vi "Create.vi"(8 "error in (no error)":errorcluster, 10 "UDP_Config":refnum<class "UDP_Config.lvclass">, 11 "UDP_Comm_Factory in":refnum<class "UDP_Comm_Factory.lvclass">) -> (0 "error out":errorcluster, 3 "UDP_Comm_Factory out":refnum<class "UDP_Comm_Factory.lvclass">)   [LabVIEW 2021, in "UDP_Comm_Factory.lvclass"]
uses:
  UDP_Comm_Factory.lvclass
  UDP_Config/UDP_Config.lvclass
  UDP_Sender/UDP_Sender.lvclass
  UDP_Receiver/UDP_Receiver.lvclass
  <vilib>/Utility/tcp.llb/UDP Multicast Write-Only Open.vi
  D:/Repository/UDP_Multicast/UDP_Comm/UDP_Comm.lvclass
  D:/Repository/UDP_Multicast/UDP_Sender/UDP_Sender.lvclass
  D:/Repository/UDP_Multicast/UDP_Receiver/UDP_Receiver.lvclass
  UDP_Comm/UDP_Comm.lvclass
panel:
  out "UDP_Comm":refnum<class "UDP_Comm.lvclass">
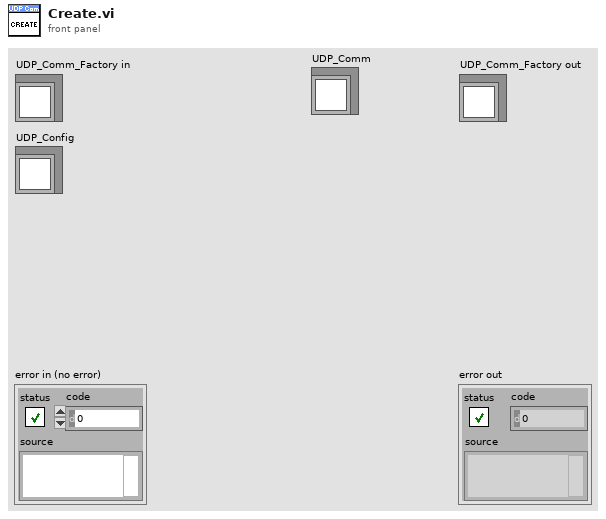
[diagram p1: front panel]
types:
  T1 = typedef "Role.ctl" = enum16{"Undefined", "Sender", "Receiver"}
  T2 = typedef "Network.ctl" = cluster{"MulticastGroup":string, "Port":u16, "LocalInterface":string, "TTL":u8}
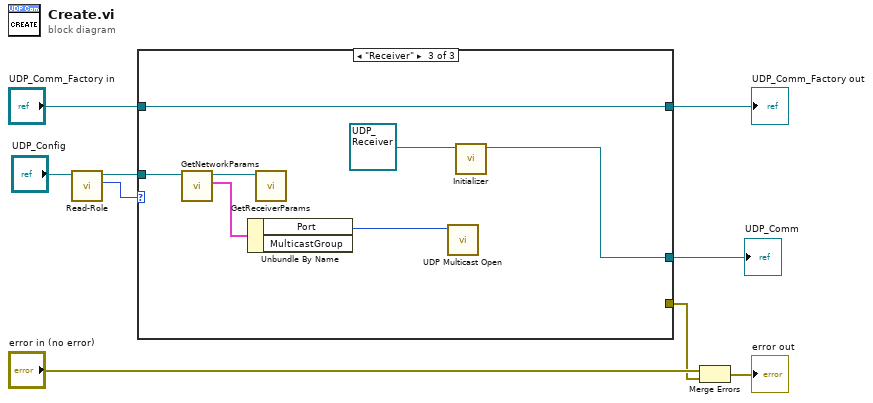
[diagram p0: block diagram]
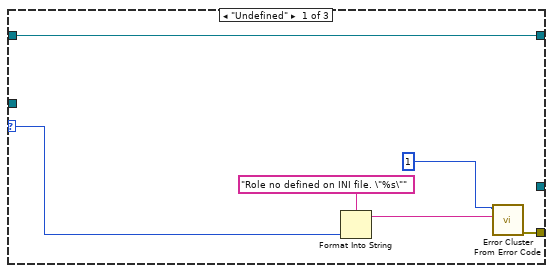
[diagram p2: hidden frame]
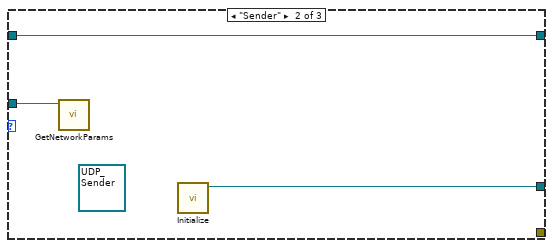
[diagram p3: hidden frame]
diagram:
  n1 = call-dynamic "Read-Role.vi"("UDP_Config in"="UDP_Config") -> ("Role"=w6:T1, "UDP_Config out"=w2:refnum<class "UDP_Config.lvclass">)  [unwired: 9 in]
  n2 = case shown="\"Receiver\"" w6 {
    selector: w6 -> [w12 _ _]
    tunnel: [w15 _ _] -> w5
    tunnel: "UDP_Comm_Factory in" -> [w10 w18 w19]
    tunnel: [w10 w18 w19] -> w3
    tunnel: [_ w16 w22] -> w1
    tunnel: w2 -> [_ w17 w25]
    frame "Undefined" {
      n3 = Format Into String(format string="Role no defined on INI file. \"%s\"", w12) -> (resulting string=w13:string)  [unwired: 2 in, 1 out]
      n4 = call <vilib>:"Error Cluster From Error Code.vi"("error message (\"\")"=w13, "error code (0)"=1 ("specific error code to clear (0: all)")) -> ("error out"=w15:errorcluster)  [unwired: 7 in]
    }
    frame "Sender" {
      (unwired) refnum<class "UDP_Sender.lvclass"> refnum ("UDP_Sender.lvclass")
      n5 = call-dynamic "GetNetworkParams.vi"("UDP_Config in"=w17) -> ()  [unwired: 9 in, 2 out]
      n6 = call-dynamic "Initialize.vi"() -> ("UDP_Sender out"=w16:refnum<class "UDP_Sender.lvclass">)  [unwired: 10 in, 1 out]
    }
    frame "Receiver" {
      n7 = call-dynamic "GetNetworkParams.vi"("UDP_Config in"=w25) -> ("Network"=w21:T2, "UDP_Config out"=w24:refnum<class "UDP_Config.lvclass">)  [unwired: 9 in]
      n8 = Unbundle By Name(w21) -> ("Port"=w20:u16)  [unwired: 1 out]
      n9 = call-dynamic "GetReceiverParams.vi"("UDP_Config in"=w24) -> ()  [unwired: 9 in, 2 out]
      n10 = call-poly <vilib>:"UDP Multicast Open.vi"("port"=w20) -> ()  [unwired: 9 in, 2 out]
      n11 = call-dynamic "Initializer.vi"("UDP_Receiver in"=refnum<class "UDP_Receiver.lvclass"> refnum ("UDP_Receiver.lvclass")) -> ("UDP_Receiver out"=w22:refnum<class "UDP_Receiver.lvclass">)  [unwired: 9 in, 1 out]
    }
  }
  "UDP_Comm_Factory out" <- w3
  "UDP_Comm" <- w1
  n12 = Merge Errors("error in (no error)", w5) -> (→"error out":errorcluster)
